vi "dealWithSNType.vi"(2 "SNXn":string="49", 3 "SNType":string="LR(YMD1)(D41)", 4 "TimeInput":timestamp=timestamp(3528403701.661259 s since 1904-01-01)) -> (0 "show_str_SNwithWholeFormat":string="LR5AN0021", 1 "legal":bool=TRUE)   [LabVIEW 2011]
panel:
  out "TimeInput-mid":timestamp=timestamp(3528403701.661259 s since 1904-01-01)
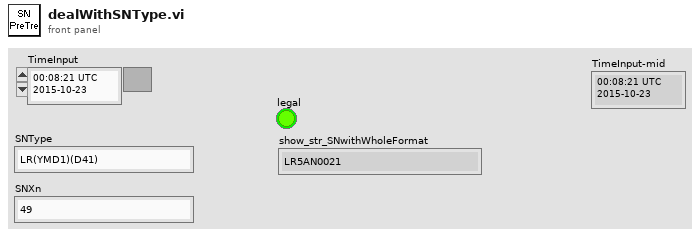
[diagram p1: front panel]
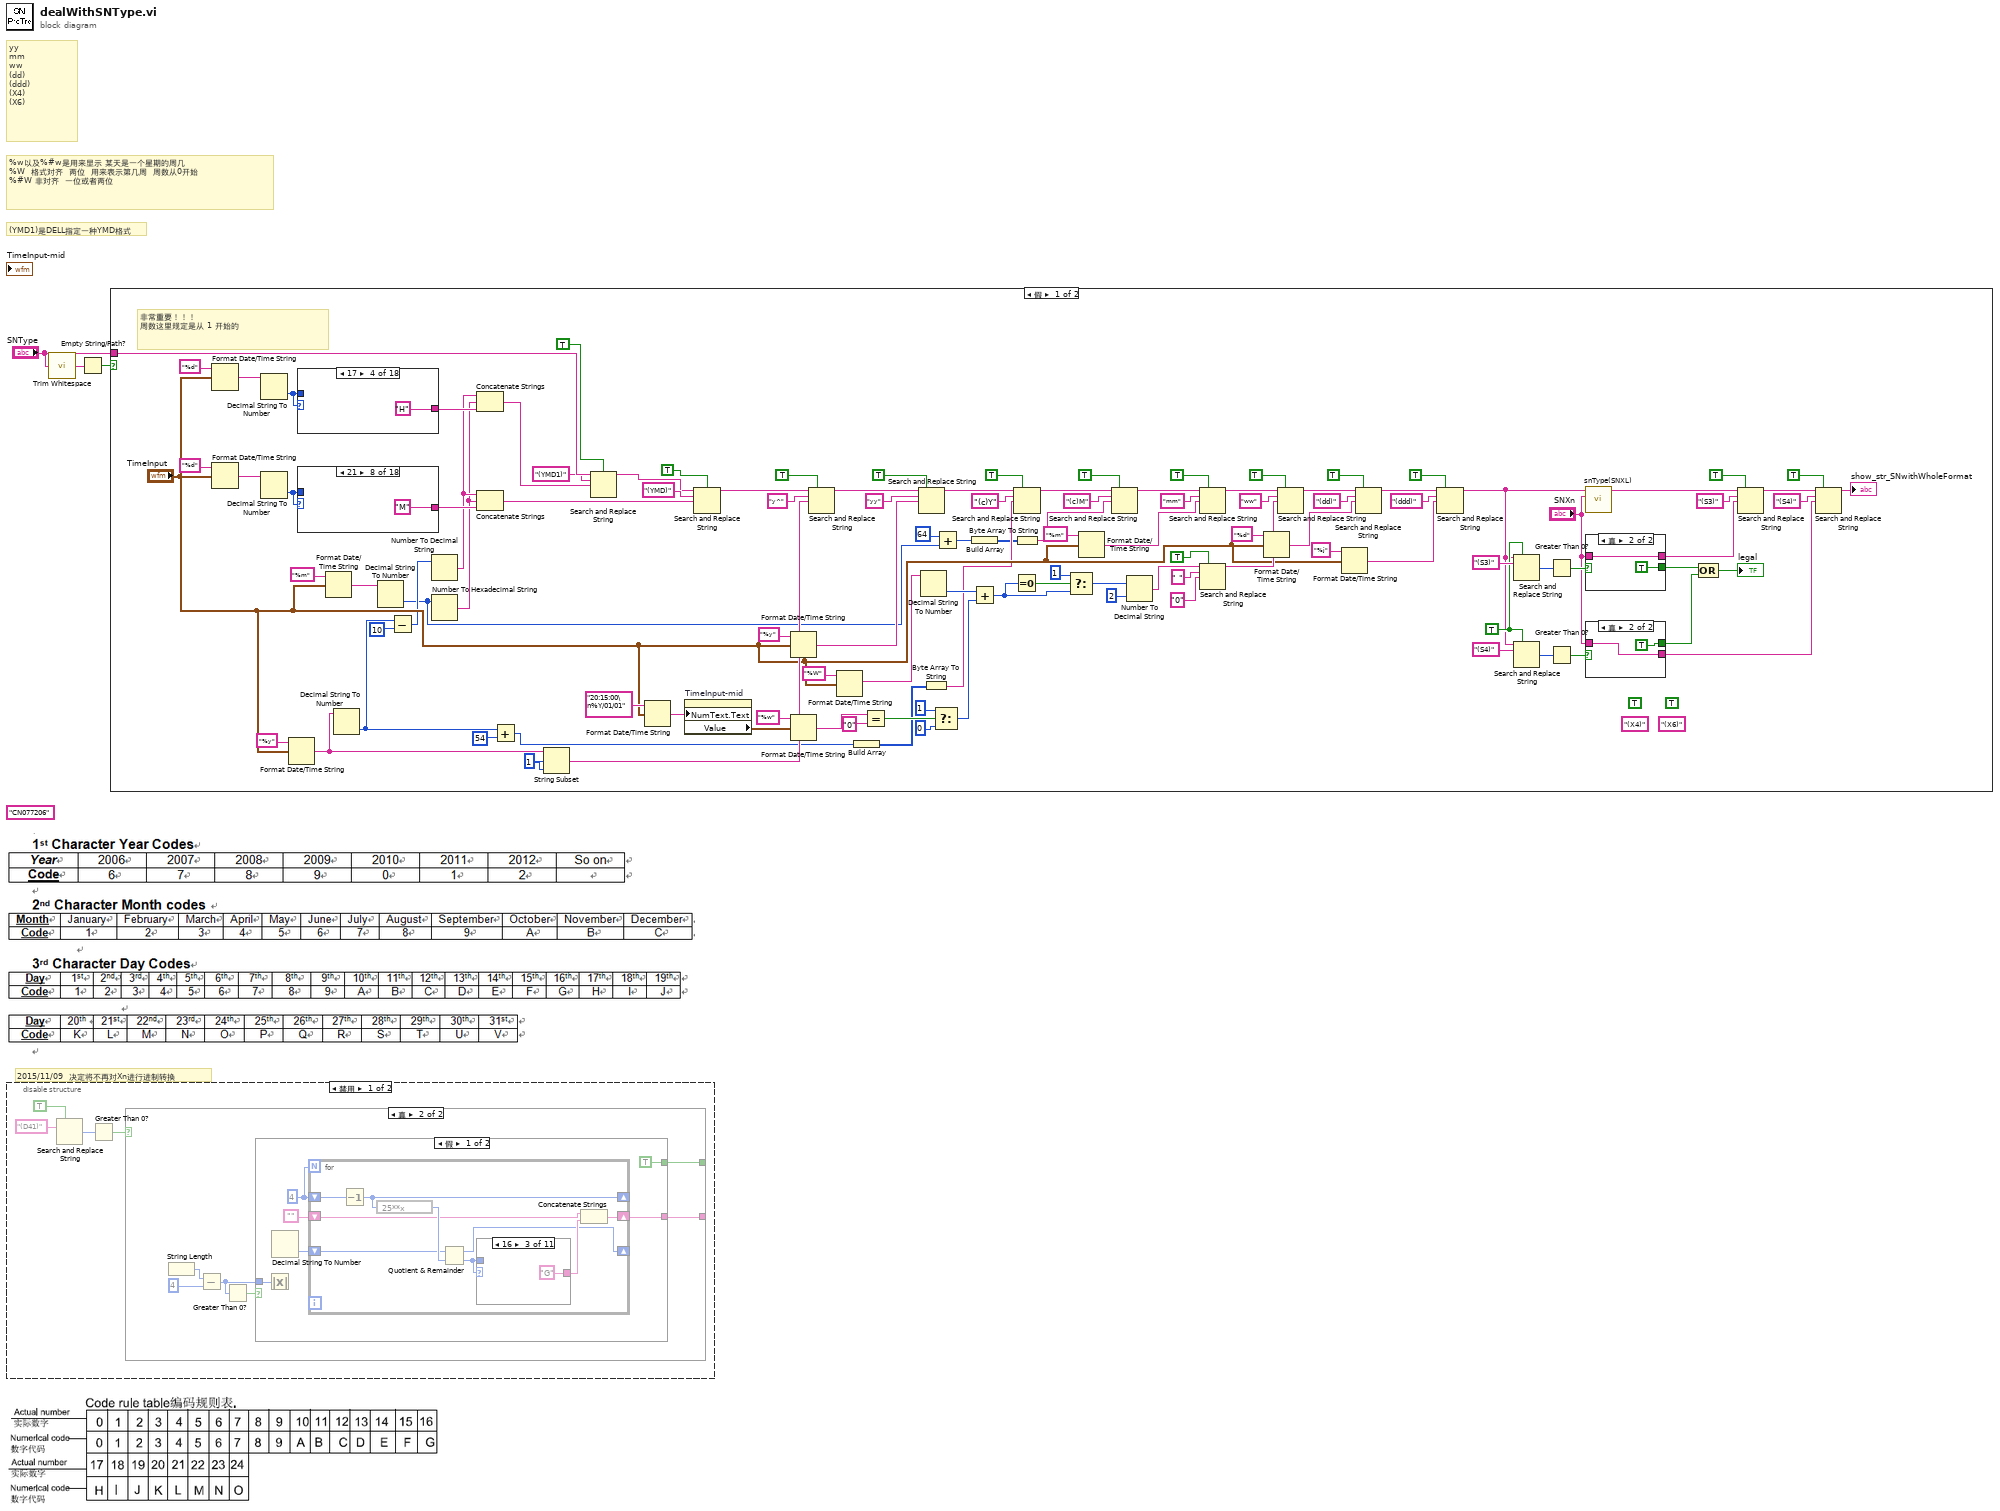
[diagram p0: block diagram]
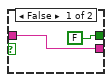
[diagram p2: hidden frame]
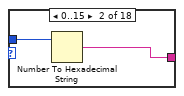
[diagram p4: hidden frame]
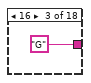
[diagram p5: hidden frame]
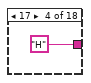
[diagram p6: hidden frame]
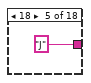
[diagram p7: hidden frame]
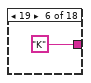
[diagram p8: hidden frame]
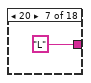
[diagram p9: hidden frame]
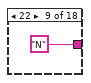
[diagram p10: hidden frame]
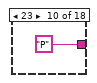
[diagram p11: hidden frame]
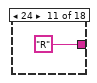
[diagram p12: hidden frame]
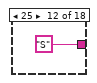
[diagram p13: hidden frame]
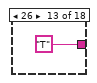
[diagram p14: hidden frame]
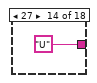
[diagram p15: hidden frame]
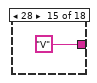
[diagram p16: hidden frame]
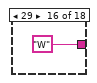
[diagram p17: hidden frame]
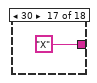
[diagram p18: hidden frame]
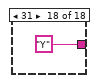
[diagram p19: hidden frame]
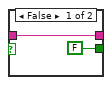
[diagram p20: hidden frame]
diagram:
  (unwired) "CN077206"
  # "2015/11/09  决定将不再对Xn进行进制转换"
  # "(YMD1)是DELL指定一种YMD格式"
  # "%w以及%#w是用来显示 某天是一个星期的周几\n%W  格式对齐  两位  用来表示第几周  周数从0开始\n%#W 非对齐  一位或者两位"
  # "yy\nmm\nww\n(dd)\n(ddd)\n(X4)\n(X6)"
  n1 = disable-structure shown="禁用" {
    frame Disabled {
      n2 = Search and Replace String(replace all?=TRUE ("替换全部？(F)"), search string="(D41)" ("搜索字符串")) -> (number of replacements=w4:i32)  [unwired: 6 in, 3 out]
      n3 = Greater Than 0?(x=w4) -> (x > 0?=w7:bool)
      n4 = case shown="真" w7 {
        tunnel: [_ w10] -> _
        tunnel: [FALSE w9] -> _
        frame False {
        }
        frame True {
          n5 = String Length() -> (length=w11:i32)  [unwired: 1 in]
          n6 = Subtract(x=w11, y=4) -> (x-y=w14:i32)
          n7 = Greater Than 0?(x=w14) -> (x > 0?=w13:bool)
          n8 = case shown="假" w13 {
            tunnel: w14 -> [w20 _]
            tunnel: [TRUE FALSE] -> w9
            tunnel: [w15 _] -> w10
            frame False {
              w17 = 4
              n9 = Absolute Value(x=w20) -> ()  [unwired: 1 out]
              n10 = Decimal String To Number() -> (number=w18:i32)  [unwired: 3 in, 1 out]
              n11 = for {
                N: w17 -> [_]
                shift-right: [w25] -> w15
                shift-left: "" -> [w26]
                shift-right: [w23] -> _
                shift-left: w17 -> [w24]
                shift-right: [w21] -> _
                shift-left: w18 -> [w22]
                n12 = Decrement(x=w24) -> (x-1=w23:i32)
                n13 = expression code="25**x"(w23) -> (w29:i32)
                n14 = Quotient & Remainder(x=w22, y=w29) -> (x-y*floor(x/y)=w21:i32, floor(x/y)=w28:i32)
                n15 = case shown="16" w28 {
                  tunnel: w28 -> [_ w31 _ _ _ _ _ _ _ _ _]
                  tunnel: [_ w30 "G" "H" "I" "J" "K" "L" "M" "N" "O"] -> w27
                  frame Default {
                  }
                  frame 0..15 {
                    n16 = Number To Hexadecimal String(2:w31) -> (0:w30:string)  [unwired: 1 in]
                  }
                  frame 16 {
                  }
                  frame 17 {
                  }
                  frame 18 {
                  }
                  frame 19 {
                  }
                  frame 20 {
                  }
                  frame 21 {
                  }
                  frame 22 {
                  }
                  frame 23 {
                  }
                  frame 24 {
                  }
                }
                n17 = Concatenate Strings(w26, w27) -> (w25:string)
              }
            }
            frame True {
              n18 = One Button Dialog(message="流水码位数和标签上选择的位数不一致！\n可能会遗失部分信息，拒绝打印！" ("消息")) -> ()  [unwired: 1 in, 1 out]
            }
          }
        }
      }
    }
    frame Enabled {
    }
  }
  n19 = call <vilib>:"Trim Whitespace.vi"("string"="SNType") -> ("trimmed string"=w2:string)  [unwired: 1 in]
  n20 = Empty String/Path?(string/path=w2) -> (empty?=w1:bool)
  n21 = case shown="假" w1 {
    tunnel: "SNType" -> [w117 _]
    frame False {
      w82 = 1 ("偏移量(0)")
      w92 = TRUE ("替换全部？(F)")
      (unwired) TRUE ("替换全部？(F)")
      (unwired) "(X6)" ("搜索字符串")
      (unwired) TRUE ("替换全部？(F)")
      (unwired) "(X4)" ("搜索字符串")
      # "非常重要！！！\n周数这里规定是从 1 开始的"
      n22 = Format Date/Time String(time format string (%c)="%d" ("时间格式字符串(%c)"), seconds (now)="TimeInput") -> (date/time string=w122:string)  [unwired: 1 in]
      n23 = Format Date/Time String(time format string (%c)="%d" ("时间格式字符串(%c)"), seconds (now)="TimeInput") -> (date/time string=w105:string)  [unwired: 1 in]
      n24 = Decimal String To Number(string=w122) -> (number=w119:i32)  [unwired: 2 in, 1 out]
      n25 = Decimal String To Number(string=w105) -> (number=w106:i32)  [unwired: 2 in, 1 out]
      n26 = Format Date/Time String(time format string (%c)="%y" ("时间格式字符串(%c)"), seconds (now)="TimeInput") -> (date/time string=w83:string)  [unwired: 1 in]
      n27 = case shown="17" w119 {
        tunnel: w119 -> [_ w183 _ _ _ _ _ _ _ _ _ _ _ _ _ _ _ _]
        tunnel: [_ w182 "G" "H" "I" "J" "K" "L" "M" "N" "O" "P" "Q" "R" "S" "T" "U" "V"] -> w118
        frame Default {
        }
        frame 0..15 {
          n28 = Number To Hexadecimal String(2:w183) -> (0:w182:string)  [unwired: 1 in]
        }
        frame 16 {
        }
        frame 17 {
        }
        frame 18 {
        }
        frame 19 {
        }
        frame 20 {
        }
        frame 21 {
        }
        frame 22 {
        }
        frame 23 {
        }
        frame 24 {
        }
        frame 25 {
        }
        frame 26 {
        }
        frame 27 {
        }
        frame 28 {
        }
        frame 29 {
        }
        frame 30 {
        }
        frame 31 {
        }
      }
      n29 = case shown="21" w106 {
        tunnel: w106 -> [_ w161 _ _ _ _ _ _ _ _ _ _ _ _ _ _ _ _]
        tunnel: [_ w160 "G" "H" "J" "K" "L" "M" "N" "P" "R" "S" "T" "U" "V" "W" "X" "Y"] -> w107
        frame Default {
        }
        frame 0..15 {
          n30 = Number To Hexadecimal String(2:w161) -> (0:w160:string)  [unwired: 1 in]
        }
        frame 16 {
        }
        frame 17 {
        }
        frame 18 {
        }
        frame 19 {
        }
        frame 20 {
        }
        frame 21 {
        }
        frame 22 {
        }
        frame 23 {
        }
        frame 24 {
        }
        frame 25 {
        }
        frame 26 {
        }
        frame 27 {
        }
        frame 28 {
        }
        frame 29 {
        }
        frame 30 {
        }
        frame 31 {
        }
      }
      n31 = Format Date/Time String(time format string (%c)="%m" ("时间格式字符串(%c)"), seconds (now)="TimeInput") -> (date/time string=w123:string)  [unwired: 1 in]
      n32 = Decimal String To Number(string=w83) -> (number=w61:i32)  [unwired: 2 in, 1 out]
      n33 = Decimal String To Number(string=w123) -> (number=w56:i32)  [unwired: 2 in, 1 out]
      n34 = Subtract(x=w61, y=10) -> (x-y=w62:i32)
      n35 = Number To Decimal String(number=w62) -> (decimal integer string=w103:string)  [unwired: 1 in]
      n36 = Number To Hexadecimal String(2:w56) -> (0:w102:string)  [unwired: 1 in]
      n37 = Concatenate Strings(w103, w102, w118) -> (w115:string)
      n38 = Concatenate Strings(w103, w102, w107) -> (w99:string)
      n39 = Add(x=w61, y=54) -> (x+y=w59:i32)
      n40 = String Subset(string=w83, offset (0)=w82, length (rest)=w82) -> (substring=w81:string)
      n41 = Search and Replace String(case sensitive?=TRUE ("忽略大小写？(F)"), input string=w117, search string="(YMD1)" ("搜索字符串"), replace string=w115) -> (result string=w100:string)  [unwired: 4 in, 3 out]
      n42 = Format Date/Time String(time format string (%c)="20:15:00\n%Y/01/01" ("时间格式字符串(%c)"), seconds (now)="TimeInput") -> (date/time string=w75:string)  [unwired: 1 in]
      n43 = property on="TimeInput-mid" class="AbsTime (严格)"("NumText.Text"=w75) -> ("Value"=w74:timestamp)  [unwired: 2 in, 2 out]
      n44 = Search and Replace String(case sensitive?=TRUE ("忽略大小写？(F)"), input string=w100, search string="(YMD)" ("搜索字符串"), replace string=w99) -> (result string=w86:string)  [unwired: 4 in, 3 out]
      n45 = Format Date/Time String(time format string (%c)="%y" ("时间格式字符串(%c)"), seconds (now)="TimeInput") -> (date/time string=w153:string)  [unwired: 1 in]
      n46 = Format Date/Time String(time format string (%c)="%w" ("时间格式字符串(%c)"), seconds (now)=w74) -> (date/time string=w72:string)  [unwired: 1 in]
      n47 = Search and Replace String(replace all?=TRUE ("替换全部？(F)"), input string=w86, search string="y^" ("搜索字符串"), replace string=w81) -> (result string=w80:string)  [unwired: 4 in, 3 out]
      n48 = Format Date/Time String(time format string (%c)="%W" ("时间格式字符串(%c)"), seconds (now)="TimeInput") -> (date/time string=w132:string)  [unwired: 1 in]
      n49 = Build Array(w59) -> (w58:i32[])
      n50 = Equal?(x=w72, y="0") -> (x = y?=w70:bool)
      n51 = Search and Replace String(replace all?=TRUE ("替换全部？(F)"), input string=w80, search string="yy" ("搜索字符串"), replace string=w153) -> (result string=w65:string)  [unwired: 4 in, 3 out]
      n52 = Decimal String To Number(string=w132) -> (number=w78:i32)  [unwired: 2 in, 1 out]
      n53 = Byte Array To String(unsigned byte array=w58) -> (string=w57:string)
      n54 = Select(t=1 ("宽度(-)"), s=w70, f=0 ("宽度(-)")) -> (s? t:f=w79:i32)
      n55 = Add(x=64, y=w56) -> (x+y=w54:i32)
      n56 = Build Array(w54) -> (w53:i32[])
      n57 = Add(x=w78, y=w79) -> (x+y=w67:i32)
      n58 = Equal To 0?(x=w67) -> (x = 0?=w69:bool)
      n59 = Search and Replace String(replace all?=TRUE ("替换全部？(F)"), input string=w65, search string="(c)Y" ("搜索字符串"), replace string=w57) -> (result string=w52:string)  [unwired: 4 in, 3 out]
      n60 = Byte Array To String(unsigned byte array=w53) -> (string=w49:string)
      n61 = Select(t=1 ("宽度(-)"), s=w69, f=w67) -> (s? t:f=w66:i32)
      n62 = Format Date/Time String(time format string (%c)="%m" ("时间格式字符串(%c)"), seconds (now)="TimeInput") -> (date/time string=w150:string)  [unwired: 1 in]
      n63 = Search and Replace String(replace all?=TRUE ("替换全部？(F)"), input string=w52, search string="(c)M" ("搜索字符串"), replace string=w49) -> (result string=w51:string)  [unwired: 4 in, 3 out]
      n64 = Number To Decimal String(number=w66, width (-)=i16 2 ("宽度(-)")) -> (decimal integer string=w130:string)
      n65 = Search and Replace String(replace all?=TRUE ("替换全部？(F)"), input string=w51, search string="mm" ("搜索字符串"), replace string=w150) -> (result string=w134:string)  [unwired: 4 in, 3 out]
      n66 = Search and Replace String(replace all?=TRUE ("替换全部？(F)"), input string=w130, search string=" " ("搜索字符串"), replace string="0" ("替换字符串(\"\")")) -> (result string=w127:string)  [unwired: 4 in, 3 out]
      n67 = Format Date/Time String(time format string (%c)="%d" ("时间格式字符串(%c)"), seconds (now)="TimeInput") -> (date/time string=w145:string)  [unwired: 1 in]
      n68 = Search and Replace String(replace all?=TRUE ("替换全部？(F)"), input string=w134, search string="ww" ("搜索字符串"), replace string=w127) -> (result string=w133:string)  [unwired: 4 in, 3 out]
      n69 = Format Date/Time String(time format string (%c)="%j" ("时间格式字符串(%c)"), seconds (now)="TimeInput") -> (date/time string=w142:string)  [unwired: 1 in]
      n70 = Search and Replace String(replace all?=TRUE ("替换全部？(F)"), input string=w133, search string="(dd)" ("搜索字符串"), replace string=w145) -> (result string=w139:string)  [unwired: 4 in, 3 out]
      n71 = Search and Replace String(replace all?=TRUE ("替换全部？(F)"), input string=w139, search string="(ddd)" ("搜索字符串"), replace string=w142) -> (result string=w45:string)  [unwired: 4 in, 3 out]
      n72 = Search and Replace String(replace all?=w92, input string=w45, search string="(S3)" ("搜索字符串")) -> (number of replacements=w113:i32)  [unwired: 5 in, 3 out]
      n73 = Search and Replace String(replace all?=w92, input string=w45, search string="(S4)" ("搜索字符串")) -> (number of replacements=w90:i32)  [unwired: 5 in, 3 out]
      n74 = Greater Than 0?(x=w113) -> (x > 0?=w112:bool)
      n75 = Greater Than 0?(x=w90) -> (x > 0?=w89:bool)
      n76 = call "snType(SNXL).vi"("SNXn"="SNXn", "SNType"=w45) -> ("show_str_SNwithWholeFormat"=w43:string)  [unwired: 9 in]
      n77 = case shown="真" w112 {
        tunnel: "SNXn" -> [w179 w181]
        tunnel: [w179 w181] -> w108
        tunnel: [FALSE TRUE] -> w111
        frame False {
        }
        frame True {
        }
      }
      n78 = case shown="真" w89 {
        tunnel: "SNXn" -> [w157 w159]
        tunnel: [w157 w159] -> w88
        tunnel: [FALSE TRUE] -> w87
        frame False {
        }
        frame True {
        }
      }
      n79 = Compound Arithmetic op=OR(w111, w87) -> (→"legal":bool)
      n80 = Search and Replace String(replace all?=TRUE ("替换全部？(F)"), input string=w43, search string="(S3)" ("搜索字符串"), replace string=w108) -> (result string=w95:string)  [unwired: 4 in, 3 out]
      n81 = Search and Replace String(replace all?=TRUE ("替换全部？(F)"), input string=w95, search string="(S4)" ("搜索字符串"), replace string=w88) -> (result string=→"show_str_SNwithWholeFormat":string)  [unwired: 4 in, 3 out]
    }
    frame True {
      n82 = local read "SNXn"() -> (w200:string)
      n83 = local write "legal"(TRUE ("legal")) -> ()
      n84 = local write "show_str_SNwithWholeFormat"(w200) -> ()
    }
  }
